vi "labview_project.vi"() -> ()   [LabVIEW 2020]
uses:
  <vilib>/MakerHub/LINX/Public/Sensors/Accelerometer/MPU60X0/DeviceAddresses.ctl
  <vilib>/MakerHub/LINX/Public/Sensors/Accelerometer/MPU60X0/Clock Source.ctl
  <vilib>/MakerHub/LINX/Public/Sensors/Accelerometer/MPU60X0/GyroFullScaleRanges.ctl
  <vilib>/Analysis/Matrix/Numeric/Conversions/Matrix To Array - RM.vi
  <vilib>/MakerHub/LINX/Public/Peripherals/PWM/PWM Set Duty Cycle N Chans.vi
  <vilib>/addons/control/pid/pid.llb/PID (DBL).vi
  <vilib>/MakerHub/LINX/Public/Utilities/Open Serial.vi
  <vilib>/MakerHub/LINX/LMH-LINX.lvlib
  <vilib>/MakerHub/LINX/Public/Sensors/Accelerometer/MPU60X0/MPU60X0.lvlib
  <vilib>/Analysis/Matrix/NI_Matrix.lvlib
  <vilib>/addons/control/pid/NI_PID_pid.lvlib
panel:
  in  "Angle":dbl
  in  "PID gains":T1={"proportional gain (Kc)"=1.0, "integral time (Ti, min)"=0.01, "derivative time (Td, min)"=0.0} {"derivative time (Td, min)" format="%.3f"; "integral time (Ti, min)" format="%.3f"; "proportional gain (Kc)" format="%.3f"}
  out "Vitesse":i16(graph)
  out "Angle":dbl(graph)
  out "pitch angle":dbl
  out "roll angle":dbl
  in  "stop":bool
  out "Gyroscope Temperature":dbl
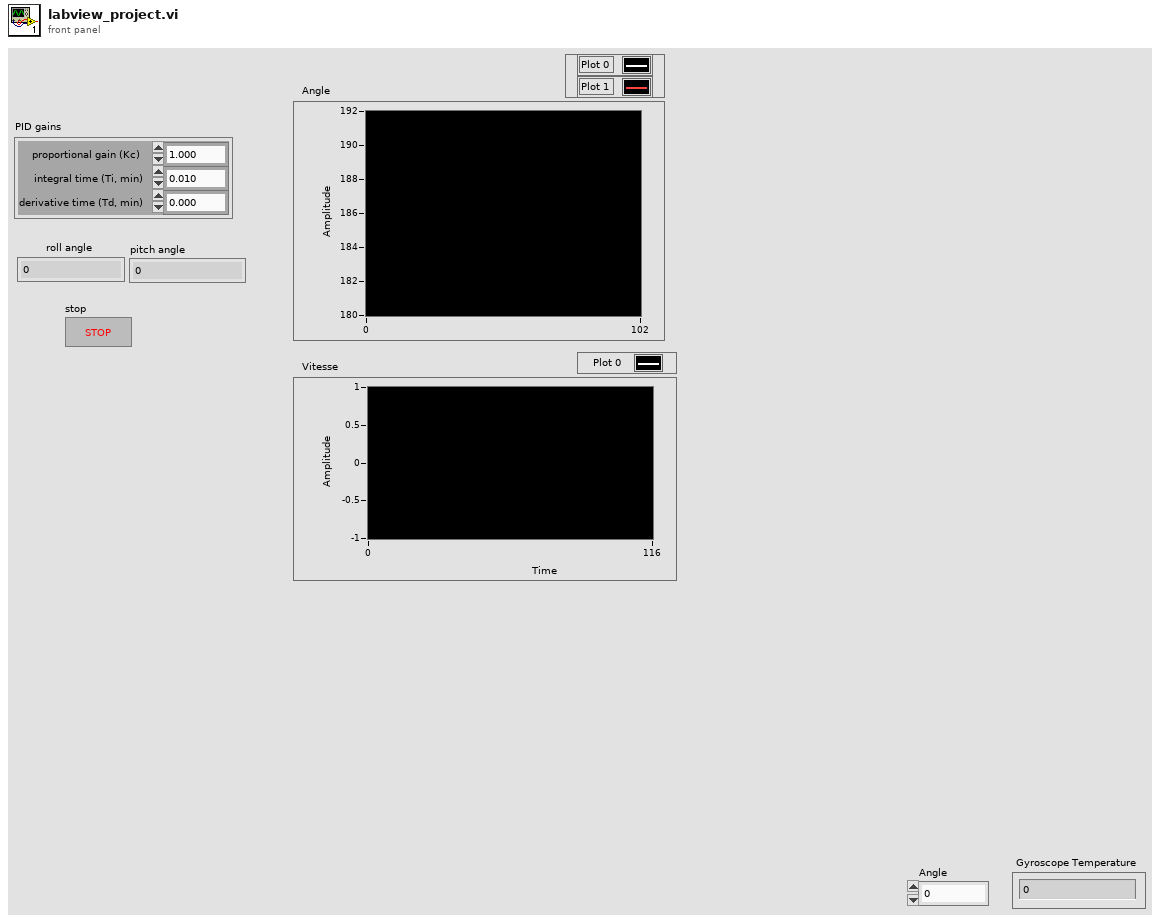
[diagram p1: front panel]
types:
  T1 = cluster{"proportional gain (Kc)":dbl, "integral time (Ti, min)":dbl, "derivative time (Td, min)":dbl}
  T2 = typedef "LMH-LINX.lvlib/MPU60X0.lvlib/GyroFullScaleRanges.ctl" = enum8{"±250 °/s", "±500 °/s", "±1000 °/s", "±2000 °/s"}
  T3 = typedef "LMH-LINX.lvlib/MPU60X0.lvlib/Clock Source.ctl" = enum8{"Internal 8MHz Osc", "PLL with X Gyro Ref", "PLL with Y Gyro Ref", "PLL with Z Gyro Ref", "PLL with ext 32.768 KHz Ref", "PLL with ext 19.2 MHz Ref", "Reserved", "Hold in reset"}
  T4 = typedef "LMH-LINX.lvlib/MPU60X0.lvlib/DeviceAddresses.ctl" = enum16{"0x68", "0x69"}
  T5 = typedef "LMH-LINX.lvlib/LINX Ref.ctl" = cluster{"IO":T6, "Interface":T7, "LINX Device Config":T8}
  T6 = typedef "LMH-LINX.lvlib/Platform.ctl" = enum16{"Remote", "Local"}
  T7 = typedef "LMH-LINX.lvlib/Interface.ctl" = enum16{"Serial", "TCP"}
  T8 = typedef "LMH-LINX.lvlib/Device.lvlib/LINX Device Config.ctl" = cluster{"Interface":T7, "COM Port":refnum<visa-resource-name>, "TCP Configuration":T9, "Device Family":u8, "Device ID":u8, "Device Name":string, "TCP Ref":refnum<k5>, "Channels":T10}
  T9 = typedef "LMH-LINX.lvlib/Device.lvlib/TCP Config.ctl" = cluster{"IP Address":string, "Port":u16}
  T10 = typedef "LMH-LINX.lvlib/Channels.ctl" = cluster{"DI":u8[], "DO":u8[], "AI":u8[], "AO":u8[], "PWM":u8[], "QE":u8[], "UART":u8[], "I2C 2":u8[], "SPI":u8[], "CAN":u8[], "Servo":u8[], "AI Ref (V)":dbl, "AI Resolution (Bits)":u8, "AO Ref (V)":dbl, "AO Resolution (Bits)":u8}
  T11 = cluster{"X Axis":i16, "Y Axis":i16, "Z Axis":i16}
  T12 = typedef "NI_Matrix.lvlib/RealMatrix.ctl" = dbl[][]
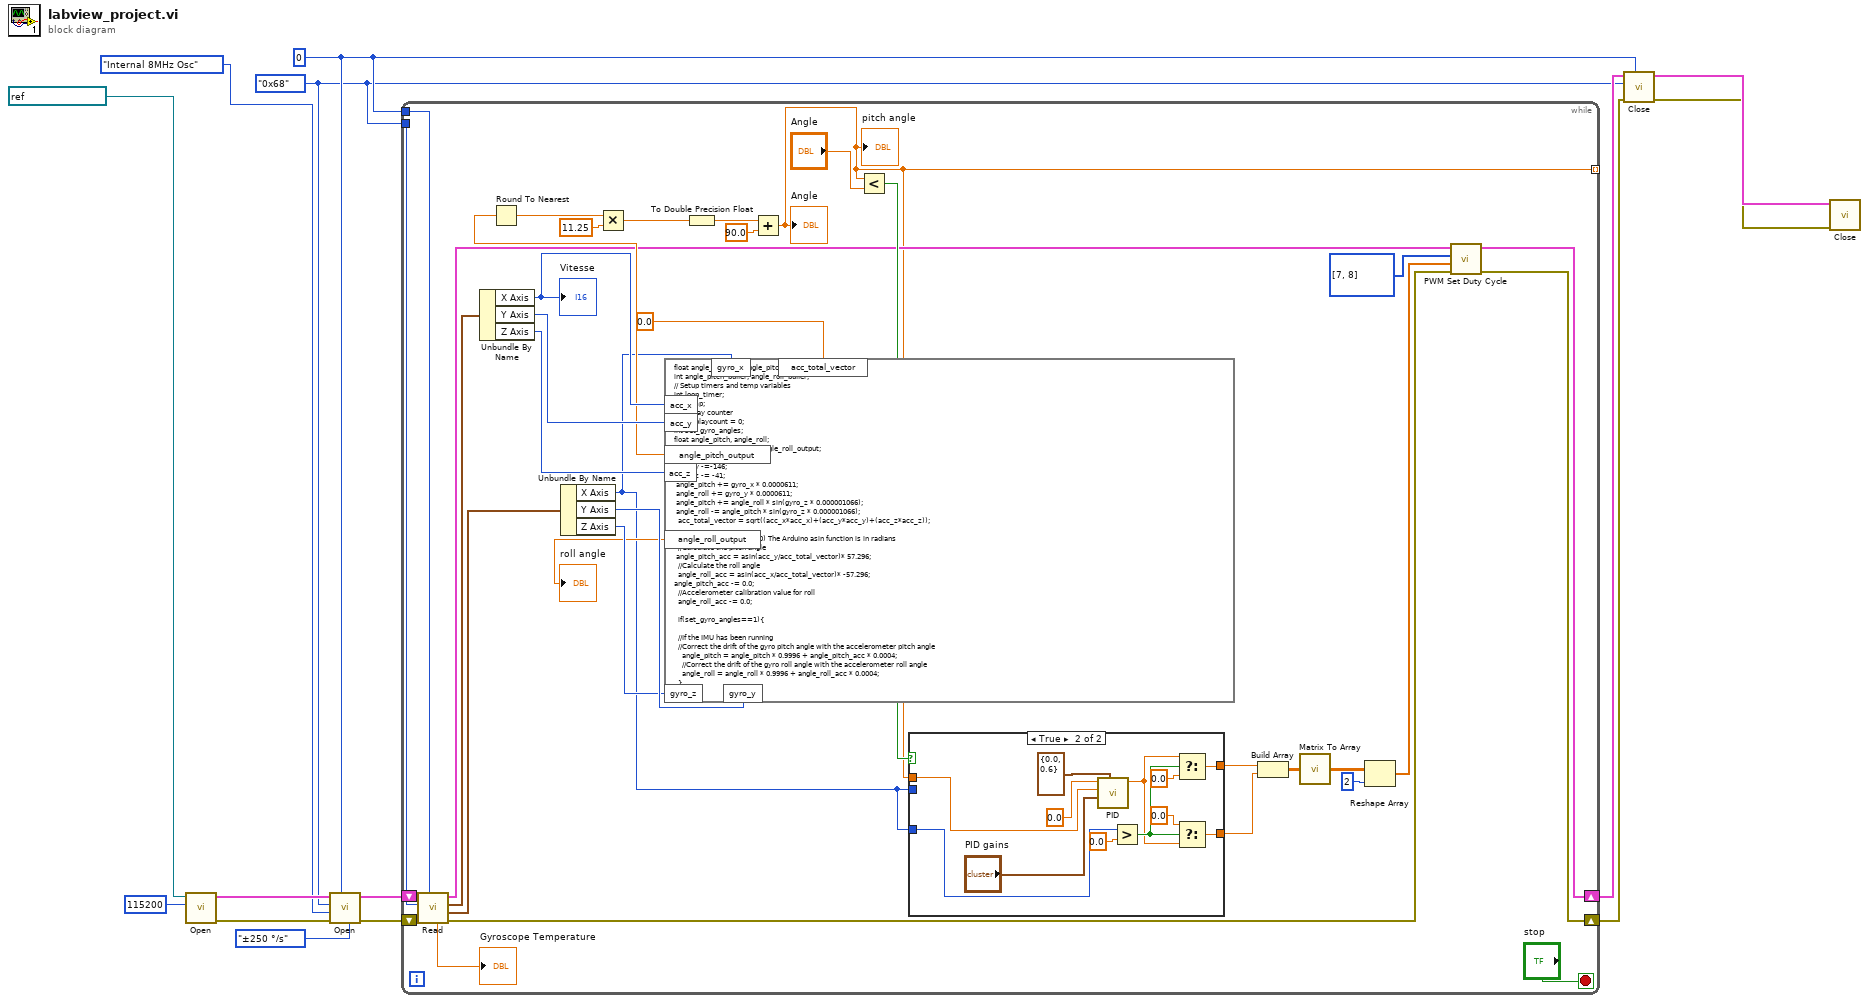
[diagram p0: block diagram]
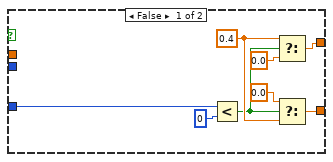
[diagram p2: hidden frame]
diagram:
  w6 = u8 0 ("I2C Channel")
  w2 = DeviceAddresses."0x68" ("I2C Slave Address")
  n1 = call-poly <vilib>:"Open.vi"("Baud Rate Override"=u32 115200, "Serial Port"=refnum<visa-resource-name> "ASRL5::INSTR") -> ("Error Out"=w10:errorcluster, "LINX Resource"=w14:T5)  [unwired: 7 in, 1 out]
  n2 = call <vilib>:"Open.vi"("Gyro Full Scale Range"=GyroFullScaleRanges."±250 °/s", "I2C Channel"=w6, "Error In"=w10, "Clock Source"=Clock_Source."Internal 8MHz Osc", "I2C Slave Address"=w2, "LINX Resource"=w14) -> ("Error Out"=w9:errorcluster, "LINX Resource"=w13:T5)  [unwired: 4 in]
  n3 = while {
    tunnel: w6 -> [w48]
    tunnel: w2 -> [w47]
    shift-right: [w29] -> w12
    shift-left: w13 -> [w50]
    shift-right: [w30] -> w8
    shift-left: w9 -> [w49]
    tunnel: [w20] -> _ mode=indexing
    stop <- "stop" stop-if-true
    n4 = call <vilib>:"Read.vi"("I2C Channel"=w48, "Error In"=w49, "I2C Slave Address"=w47, "LINX Resource"=w50) -> ("Error Out"=w32:errorcluster, "Gyro  Data (dps)"=w43:T11, "Acceleration Data (g)"=w44:T11, "LINX Resource"=w31:T5, "Temperature (°C)"=→"Gyroscope Temperature":dbl)  [unwired: 3 in]
    n5 = Unbundle By Name(w44) -> ("X Axis"=w36:i16, "Y Axis"=w39:i16, "Z Axis"=w38:i16)
    "Vitesse" <- w36
    n6 = Unbundle By Name(w43) -> ("X Axis"=w16:i16, "Y Axis"=w42:i16, "Z Axis"=w41:i16)
    n7 = formula code="float angle_roll_acc, angle_pitch_acc; \nint angle_pitch_buffer, angle_roll_buffer;\n// Setup timers and temp variables\nint loop_timer;\nint temp;\n// Display counter\nint displaycount = 0;\nint set_gyro_angles;\nfloat angle_pitch, angle_roll;\nfloat angle_pitch_output, angle_roll_output;\ngyro_x -= -121;                                                \n gyro_y -=-146;                                                \n gyro_z -= -41;                                                \n angle_pitch += gyro_x * 0.0000611;  \n angle_roll += gyro_y * 0.0000611; \n angle_pitch += angle_roll * sin(gyro_z * 0.000001066);             \n angle_roll -= angle_pitch * sin(gyro_z * 0.000001066);        \n  acc_total_vector = sqrt((acc_x*acc_x)+(acc_y*acc_y)+(acc_z*acc_z)); \n   \n  //57.296 = 1 / (3.142 / 180) The Arduino asin function is in radians\n  //Calculate the pitch angle\n angle_pitch_acc = asin(acc_y/acc_total_vector)* 57.296; \n  //Calculate the roll angle      \n  angle_roll_acc = asin(acc_x/acc_total_vector)* -57.296;                 \nangle_pitch_acc -= 0.0;\n  //Accelerometer calibration value for roll                                              \n  angle_roll_acc -= 0.0;                                               \n \n  if(set_gyro_angles==1){ \n  \n  //If the IMU has been running \n  //Correct the drift of the gyro pitch angle with the accelerometer pitch angle                      \n    angle_pitch = angle_pitch * 0.9996 + angle_pitch_acc * 0.0004; \n    //Correct the drift of the gyro roll angle with the accelerometer roll angle    \n    angle_roll = angle_roll * 0.9996 + angle_roll_acc * 0.0004;        \n  }\n  else{ \n    //IMU has just started  \n    //Set the gyro pitch angle equal to the accelerometer pitch angle                                                           \n    angle_pitch = angle_pitch_acc;\n    //Set the gyro roll angle equal to the accelerometer roll angle                                       \n    angle_roll = angle_roll_acc;\n    //Set the IMU started flag                                       \n    set_gyro_angles = 1;                                            \n  }\n  \n //To dampen the pitch and roll angles a complementary filter is used\n //Take 90% of the output pitch value and add 10% of the raw pitch value\nangle_pitch_output =angle_pitch_output * 0.9 + angle_pitch * 0.1; \n//Take 90% of the output roll value and add 10% of the raw roll value \nangle_roll_output = angle_roll_output * 0.9 + angle_roll * 0.1;\n//angle_pitch_output=11,25*angle_pitch_output; \n//angle_roll_output=11,25*angle_roll_output; \n\n//Wait until the loop_timer reaches 4000us (250Hz) before starting the next loop  \n   \n// Increment the display counter\ndisplaycount = displaycount +1;"("gyro_x"=w16, "gyro_y"=w42, "gyro_z"=w41, "acc_x"=w36, "acc_y"=w39, "acc_z"=w38, "acc_total_vector"=0.0) -> ("angle_pitch_output"=w34:dbl, "angle_roll_output"=→"roll angle":dbl)
    n8 = Round To Nearest(number=w34) -> (nearest integer value=w35:dbl)
    n9 = Multiply(x=w35, y=11.25) -> (x*y=w22:dbl)
    n10 = To Double Precision Float(number=w22) -> (double precision float=w19:dbl)
    n11 = Add(x=w19, y=90.0) -> (x+y=w20:dbl)
    "pitch angle" <- w20
    "Angle" <- w20
    n12 = Less?(x=w20, y="Angle") -> (x < y?=w33:bool)
    n13 = case shown="True" w33 {
      tunnel: w20 -> [_ w63]
      tunnel: w16 -> [_ _]
      tunnel: [w54 w68] -> w18
      tunnel: [w55 w67] -> w17
      tunnel: w16 -> [w53 w65]
      frame False {
        w58 = 0.4
        n14 = Less?(x=w53, y=i16 0) -> (x < y?=w51:bool)
        n15 = Select(t=w58, s=w51, f=0.0) -> (s? t:f=w55:dbl)
        n16 = Select(t=0.0, s=w51, f=w58) -> (s? t:f=w54:dbl)
      }
      frame True {
        n17 = call-poly <vilib>:"PID.vi"("output range"=cluster{"output high":dbl, "output low":dbl} {"output high"=0.0, "output low"=0.6}, "PID gains"="PID gains", "process variable"=w63, "setpoint"=0.0) -> ("output"=w59:dbl)  [unwired: 6 in, 1 out]
        n18 = Greater?(x=w65, y=0.0) -> (0:w60:bool)
        n19 = Select(t=w59, s=w60, f=0.0) -> (s? t:f=w67:dbl)
        n20 = Select(t=0.0, s=w60, f=w59) -> (s? t:f=w68:dbl)
      }
    }
    n21 = Build Array(w17, w18) -> (w26:T12)
    n22 = call-poly <vilib>:"Matrix To Array.vi"("Real Matrix"=w26) -> ("Real 2D Array"=w27:dbl[][])
    n23 = Reshape Array(w27, 2 ("dimension size")) -> (w24:dbl[])
    n24 = call-poly <vilib>:"PWM Set Duty Cycle.vi"("Error In"=w32, "Duty Cycles"=w24, "PWM Channels"=u8[] [7, 8], "LINX Resource"=w31) -> ("Error Out"=w30:errorcluster, "LINX Resource"=w29:T5)  [unwired: 6 in]
  }
  n25 = call <vilib>:"Close.vi"("I2C Channel (0)"=w6, "Error In"=w8, "I2C Slave Address (0)"=w2, "LINX Resource"=w12) -> ("Error Out"=w7:errorcluster, "LINX Resource"=w11:T5)  [unwired: 6 in]
  n26 = call <vilib>:"Close.vi"("Error In"=w7, "LINX Resource"=w11) -> ()  [unwired: 9 in, 1 out]
